vi "test-delete this.vi"() -> ()   [LabVIEW 2018]
uses:
  Classes/database.lvclass
panel:
  out "data 2":string
  out "data":variant[][](array[variant])
  out "error out":errorcluster
  out "database out":refnum<class "database.lvclass">
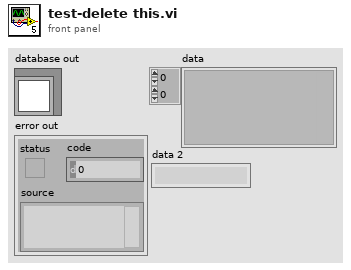
[diagram p1: front panel]
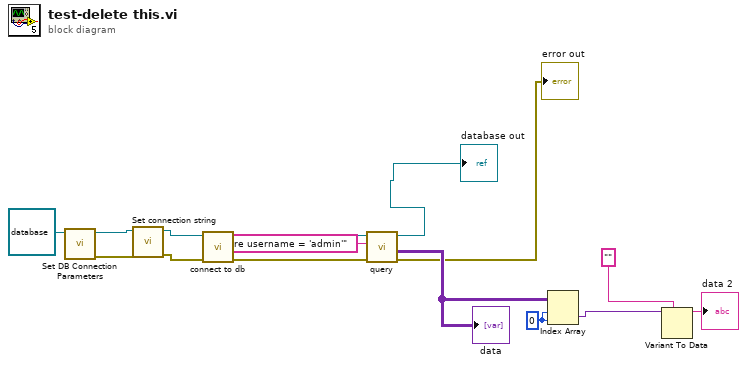
[diagram p0: block diagram]
diagram:
  w13 = 0 ("disabled index (col)")
  n1 = call-dynamic "Set DB Connection Parameters.vi"("database in"=refnum<class "database.lvclass"> refnum) -> ("error out"=w7:errorcluster, "database out"=w9:refnum<class "database.lvclass">)  [unwired: 9 in]
  n2 = call-dynamic "Set connection string.vi"("error in (no error)"=w7, "database in"=w9) -> ("error out"=w6:errorcluster, "database out"=w8:refnum<class "database.lvclass">)  [unwired: 8 in]
  n3 = call-dynamic "connect to db.vi"("error in (no error)"=w6, "database in"=w8) -> ("error out"=w3:errorcluster, "database out"=w4:refnum<class "database.lvclass">)  [unwired: 8 in]
  n4 = call-dynamic "query.vi"("error in (no error)"=w3, "condition"="where username = 'admin'", "database in"=w4) -> ("error out"=→"error out":errorcluster, "data"=w14:variant[][], "database out"=→"database out":refnum<class "database.lvclass">)  [unwired: 6 in]
  "data" <- w14
  n5 = Index Array(array=w14, index (row)=w13, index (col)=w13) -> (element=w12:variant)
  n6 = Variant To Data(type="" ("condition"), Variant=w12) -> (data=→"data 2":string)  [unwired: 1 in, 1 out]
